vi "StageMoveDiscrete.vi"(6 "time delay before acquisition (ms)":u32=1500, 8 "error in (no error)":errorcluster, 9 "acquire?":bool, 11 "Microscope in":refnum<class "Microscope.lvclass">) -> (0 "error out":errorcluster, 3 "Microscope out":refnum<class "Microscope.lvclass">)   [LabVIEW 2012, in "Microscope.lvclass"]
uses:
  classes/Microscope.lvclass
  classes/Microscope.lvclass/Microscope.ctl
  variables/GlobalUI.vi
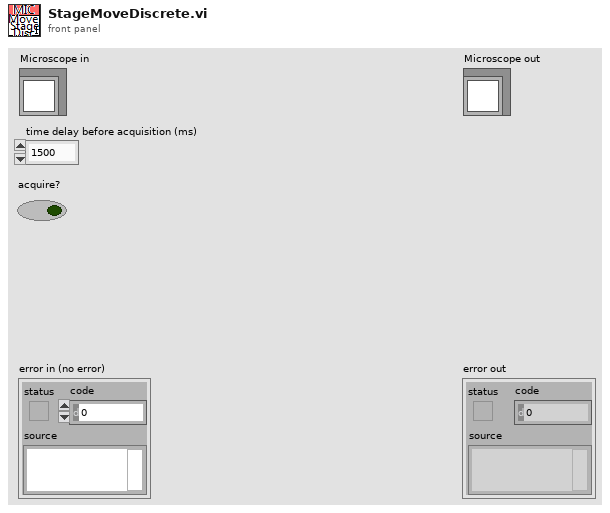
[diagram p1: front panel]
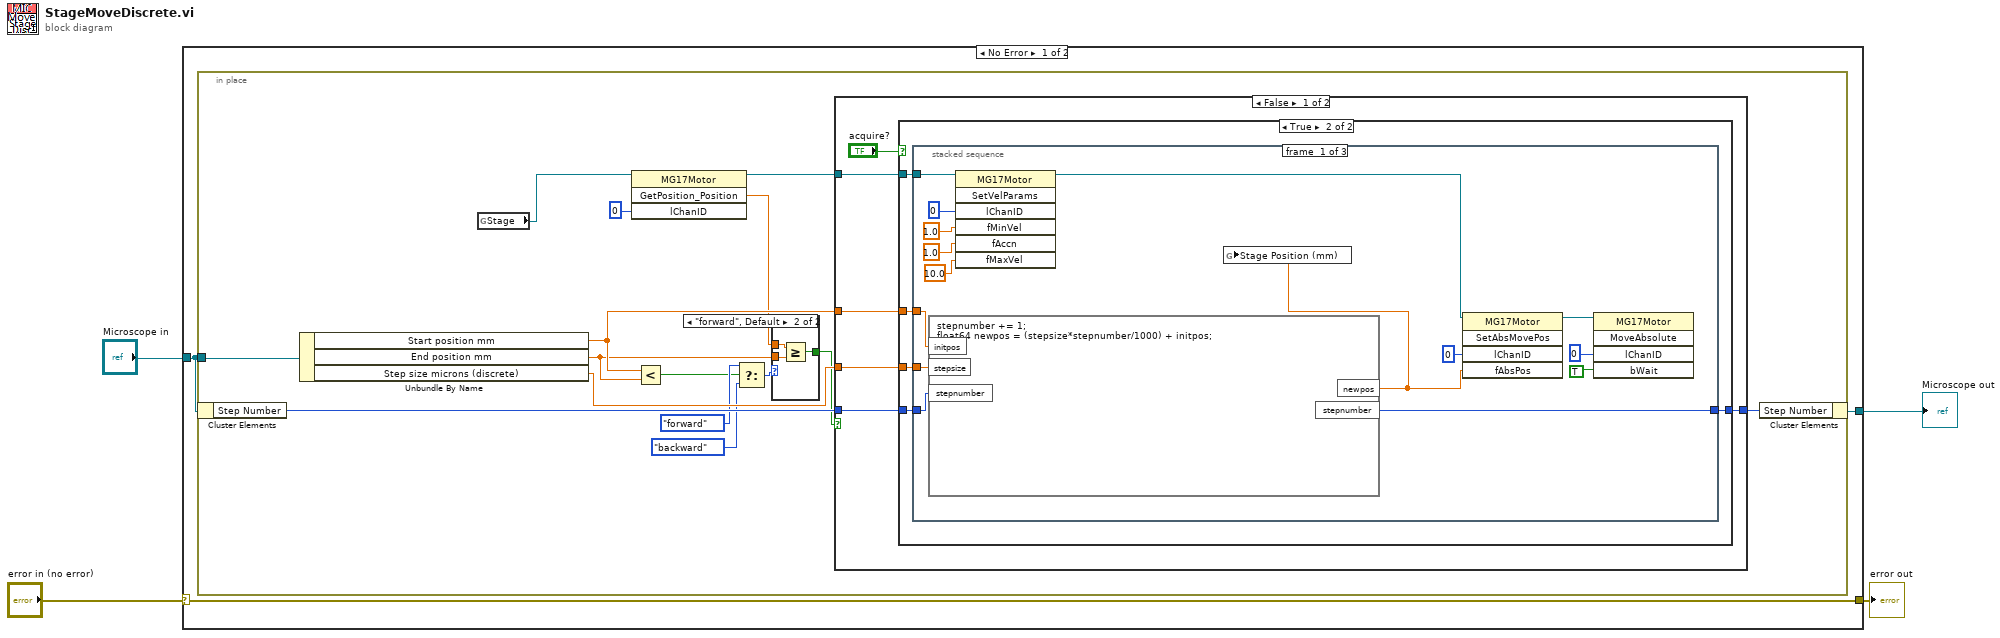
[diagram p0: block diagram]
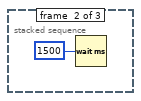
[diagram p3: hidden frame]
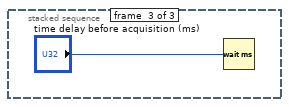
[diagram p4: hidden frame]
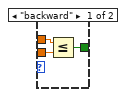
[diagram p6: hidden frame]
diagram:
  n1 = case shown="No Error" "error in (no error)" {
    selector: "error in (no error)" -> [w7 w60]
    tunnel: [w7 w60] -> w3
    tunnel: [w5 w59] -> w1
    tunnel: "Microscope in" -> [w6 w59]
    frame No Error {
      n2 = in-place {
        in-place-border: w6 -> [w9]
        n3 = in-place-cluster #1(w6) -> ("Step Number"=w19:i32)
        n4 = Unbundle By Name(w9) -> ("Start position mm"=w22:dbl, "End position mm"=w21:dbl, "Step size microns (discrete)"=w20:dbl)
        n5 = global read "GlobalUI.vi" "Stage"() -> (w8:refnum<k7>)
        n6 = invoke class="MG17Motor" method="GetPosition_Position"(reference=w8, "lChanID"=0) -> (reference out=w14:refnum<k7>, "GetPosition_Position"=w15:sgl)  [unwired: 2 in, 2 out]
        n7 = Less?(x=w22, y=w21) -> (x < y?=w12:bool)
        n8 = Select(t=enum16{"", "forward", "backward"}."forward", s=w12, f=enum16{"", "forward", "backward"}."backward") -> (s? t:f=w17:enum16{"", "forward", "backward"})
        n9 = case shown="\"forward\", Default" w17 {
          tunnel: [w55 w58] -> w11
          tunnel: w15 -> [w54 w57]
          tunnel: w21 -> [w53 w56]
          frame "backward" {
            n10 = Less Or Equal?(x=w54, y=w53) -> (x <= y?=w55:bool)
          }
          frame "forward", Default {
            n11 = Greater Or Equal?(x=w57, y=w56) -> (x >= y?=w58:bool)
          }
        }
        n12 = case shown="False" w11 {
          tunnel: w14 -> [w28 _]
          tunnel: [w26 w52] -> w10
          tunnel: w20 -> [w25 _]
          tunnel: w19 -> [w24 w52]
          tunnel: w22 -> [w23 _]
          frame False {
            n13 = case shown="True" "acquire?" {
              tunnel: w28 -> [_ w34]
              tunnel: [w29 w33] -> w26
              tunnel: w25 -> [_ w32]
              tunnel: w24 -> [w29 w31]
              tunnel: w23 -> [_ w30]
              frame False {
              }
              frame True {
                n14 = stacked-sequence {
                  tunnel: w34 -> [w40 _ _]
                  tunnel: [w45 _ _] -> w33
                  tunnel: w32 -> [w38 _ _]
                  tunnel: w31 -> [w37 _ _]
                  tunnel: w30 -> [w36 _ _]
                  frame #0 {
                    n15 = formula code="stepnumber += 1;\nfloat64 newpos = (stepsize*stepnumber/1000) + initpos;"("stepsize"=w38, "stepnumber"=w37, "initpos"=w36) -> ("stepnumber"=w45:i32, "newpos"=w35:dbl)
                    n16 = invoke class="MG17Motor" method="SetVelParams"(reference=w40, "lChanID"=0, "fMinVel"=sgl 1.0, "fAccn"=sgl 1.0, "fMaxVel"=sgl 10.0) -> (reference out=w39:refnum<k7>)  [unwired: 2 in, 6 out]
                    n17 = global write "GlobalUI.vi" "Stage Position (mm)"(w35) -> ()
                    n18 = invoke class="MG17Motor" method="SetAbsMovePos"(reference=w39, "lChanID"=0, "fAbsPos"=w35) -> (reference out=w47:refnum<k7>)  [unwired: 2 in, 4 out]
                    n19 = invoke class="MG17Motor" method="MoveAbsolute"(reference=w47, "lChanID"=0, "bWait"=TRUE) -> ()  [unwired: 2 in, 5 out]
                  }
                  frame #1 {
                    n20 = Wait (ms)(milliseconds to wait=u32 1500) -> ()  [unwired: 1 out]
                  }
                  frame #2 {
                    n21 = Wait (ms)(milliseconds to wait="time delay before acquisition (ms)") -> ()  [unwired: 1 out]
                  }
                }
              }
            }
          }
          frame True {
          }
        }
        n22 = in-place-cluster #1("Step Number"=w10) -> (w5:refnum<class "Microscope.lvclass">)
      }
    }
    frame Error {
    }
  }
  "error out" <- w3
  "Microscope out" <- w1
